vi "Description.vi"(8 "error in (no error)":errorcluster, 11 "String Input Matching Comparator in":refnum<class "Matching String Input Comparator.lvclass">) -> (0 "error out":errorcluster, 2 "Description":string)   [LabVIEW 2020, in "Matching String Input Comparator.lvclass"]
uses:
  Matching String Input Comparator.lvclass
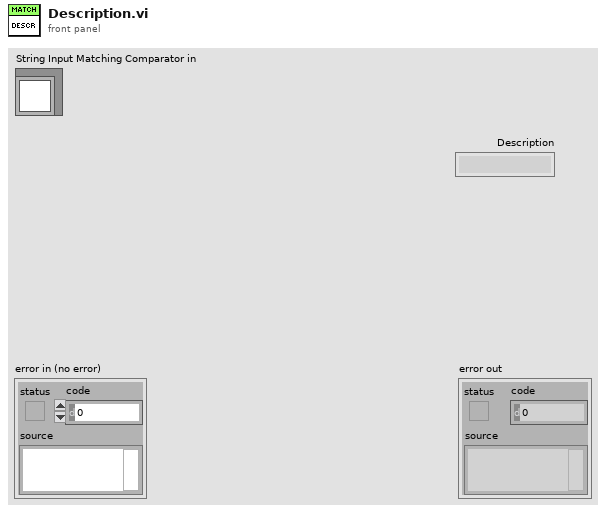
[diagram p1: front panel]
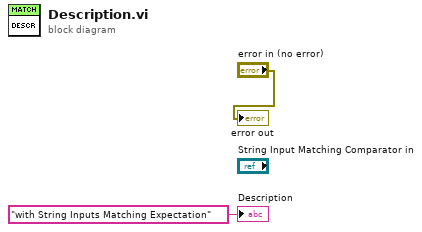
[diagram p0: block diagram]
diagram:
  "error out" <- "error in (no error)"
  "Description" <- "with String Inputs Matching Expectation" ("Description")
